vi "MMEM_MOVE.vi"(0 "VISA IN":refnum<visa-resource-name>, 1 "Tgt":string, 5 "error in":errorcluster, 7 "Src":string) -> (14 "VISA Out":refnum<visa-resource-name>, 19 "error out":errorcluster)   [LabVIEW 2018, in "PNA-X.lvlib"]
doc: "MMEMory:MOVE <file1>,<file2> \n1611\n\n(Write-only) Renames <file1> to <file2>. File extensions must be specified. \nParameters \n<file1> String - Name of the file to be renamed. See Specifying Path Names \n<file2> String - Name of the new file. \nExamples MMEM:MOVE 'MyFile.cst','YourFile.cst' \nQuery Syntax Not applicable \nDefault Not applicable"
uses:
  PNA-X.lvlib
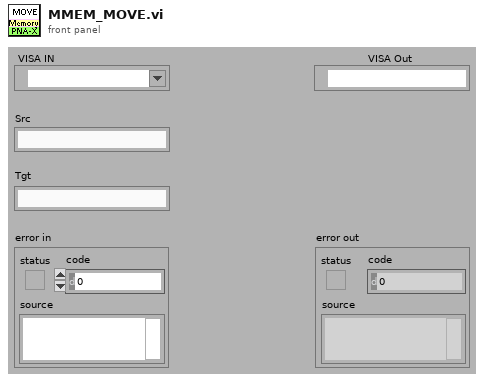
[diagram p1: front panel]
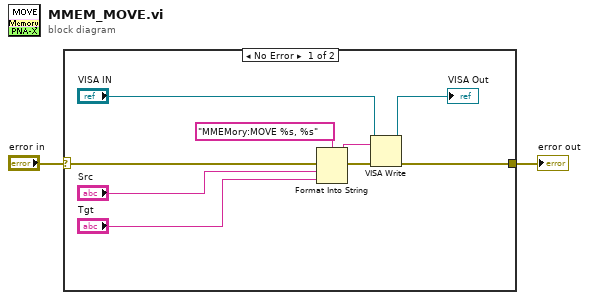
[diagram p0: block diagram]
diagram:
  n1 = case shown="No Error" "error in" {
    selector: "error in" -> [w11 w12]
    tunnel: [w6 w12] -> w1
    frame No Error {
      n2 = Format Into String(format string="MMEMory:MOVE %s, %s" ("Cmdline"), error in=w11, "Src", "Tgt") -> (resulting string=w9:string, error out=w10:errorcluster)  [unwired: 1 in]
      n3 = VISA Write(VISA resource name="VISA IN", write buffer=w9, error in (no error)=w10) -> (VISA resource name out=→"VISA Out":refnum<visa-resource-name>, error out=w6:errorcluster)  [unwired: 1 out]
    }
    frame Error {
    }
  }
  "error out" <- w1
